vi "CC Script Check For Slit.vi"(8 "error in (no error)":errorcluster, 11 "Script":T1[](array[typedef])) -> (0 "error out":errorcluster, 3 "At Slit?":bool)   [LabVIEW 2024]
uses:
  typedefs/CC Script Step.ctl
  typedefs/CC enum Script Action.ctl
  Filter Wheel/FW cmd Q Move Parameters.ctl
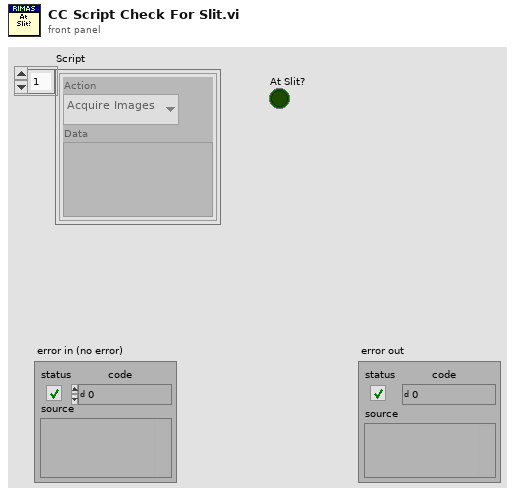
[diagram p1: front panel]
types:
  T1 = typedef "CC Script Step.ctl" = cluster{"Action":T2, "Data":variant}
  T2 = typedef "CC enum Script Action.ctl" = enum16{"Noop", "Define Object", "Define Exposure", "Define Dithering", "Acquire Images", "Set Filter Wheel", "Telescope Home", "Telescope Move", "Telescope RA DEC", "Focus Move Relative", "Focus Move Absolute", "Focus Set Home", "Macro", "Pause", "Ask User", "Define Random Dither", "CmdLine", "Outlet"}
  T3 = typedef "FW cmd Q Move Parameters.ctl" = cluster{"Wheel ID":i32, "Position":i32}
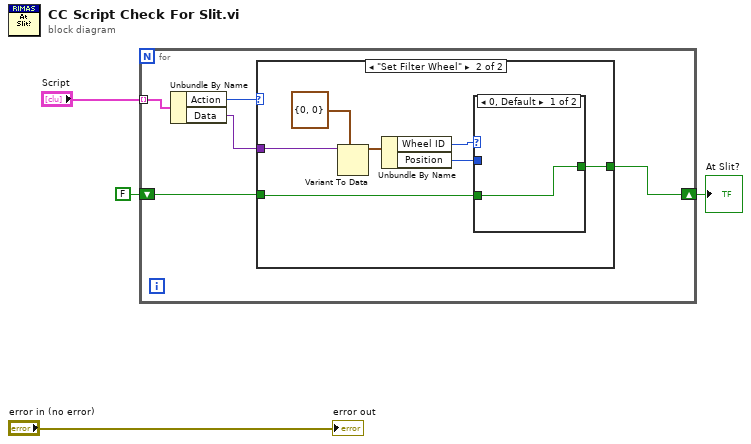
[diagram p0: block diagram]
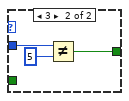
[diagram p3: hidden frame]
diagram:
  n1 = for {
    tunnel: "Script" -> [w9] mode=indexing
    shift-right: [w6] -> w1
    shift-left: FALSE -> [w5]
    n2 = Unbundle By Name(w9) -> ("Action"=w8:T2, "Data"=w7:variant)
    n3 = case shown="\"Set Filter Wheel\"" w8 {
      tunnel: w7 -> [_ w16]
      tunnel: [w10 w12] -> w6
      tunnel: w5 -> [w10 w11]
      frame "Noop", Default {
      }
      frame "Set Filter Wheel" {
        n4 = Variant To Data(type=T3 {"Wheel ID"=0, "Position"=0}, Variant=w16) -> (data=w15:T3)  [unwired: 1 in, 1 out]
        n5 = Unbundle By Name(w15) -> ("Wheel ID"=w14:i32, "Position"=w13:i32)
        n6 = case shown="0, Default" w14 {
          tunnel: w13 -> [_ w21]
          tunnel: [w18 w19] -> w12
          tunnel: w11 -> [w18 _]
          frame 0, Default {
          }
          frame 3 {
            n7 = Not Equal?(x=w21, y=5) -> (x != y?=w19:bool)
          }
        }
      }
    }
  }
  "At Slit?" <- w1
  "error out" <- "error in (no error)"
